vi "Update Watchdog Status Core.vi"(8 "Error In":errorcluster, 10 "watchdog status":T1, 11 "CS++RTMainActor in":refnum<class "CS++RTMainActor.lvclass">) -> (0 "Error Out":errorcluster, 3 "CS++RTMainActor out":refnum<class "CS++RTMainActor.lvclass">)   [LabVIEW 2016, in "CS++RTMain.lvlib" / "CS++RTMainActor.lvclass"]
doc: "Update watchdog status.\n\n<b>Derived classes should override this VI to deal with watchdog status changes.</b>"
uses:
  CS++RTMain/CS++RTMainActor.lvclass
  <vilib>/RTwatchdog.llb/Watchdog status enum.ctl
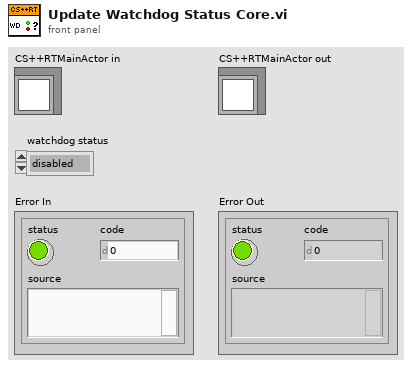
[diagram p1: front panel]
types:
  T1 = typedef "Watchdog status enum.ctl" = enum16{"disabled", "expired", "running"}
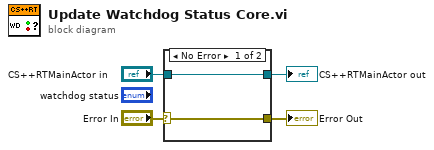
[diagram p0: block diagram]
diagram:
  n1 = case shown="No Error" "Error In" {
    selector: "Error In" -> [w5 w8]
    tunnel: [w5 w8] -> w3
    tunnel: [w6 w7] -> w1
    tunnel: "CS++RTMainActor in" -> [w6 w7]
    frame No Error {
    }
    frame Error {
    }
  }
  "Error Out" <- w3
  "CS++RTMainActor out" <- w1
